vi "Sine Wave Generation.vi"() -> ()   [LabVIEW 2022 SP3]
uses:
  <instrlib>/niUSRP/niUSRP Write Tx Data (CDB).vi
panel:
  in  "Waveform size":i32
  out "coerced gain":dbl format="%#_6f"
  out "coerced carrier frequency":dbl=100000.0 format="%#_6p"
  out "coerced IQ rate":dbl=100000.0 format="%#_6p"
  in  "active antenna 2":string
  in  "gain (dB)":dbl
  in  "?":bool
  in  "frequency (Hz)":dbl
  in  "IQ rate (S/s)":dbl
  in  "USRP IP Address":refnum<k15>
  out "error out":errorcluster
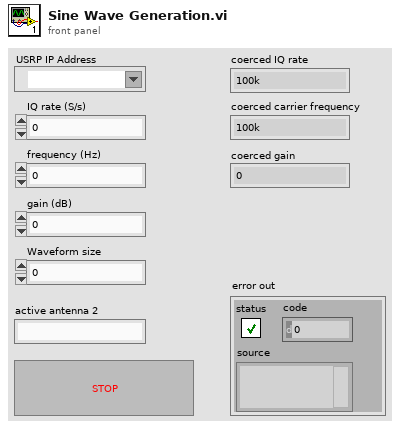
[diagram p1: front panel]
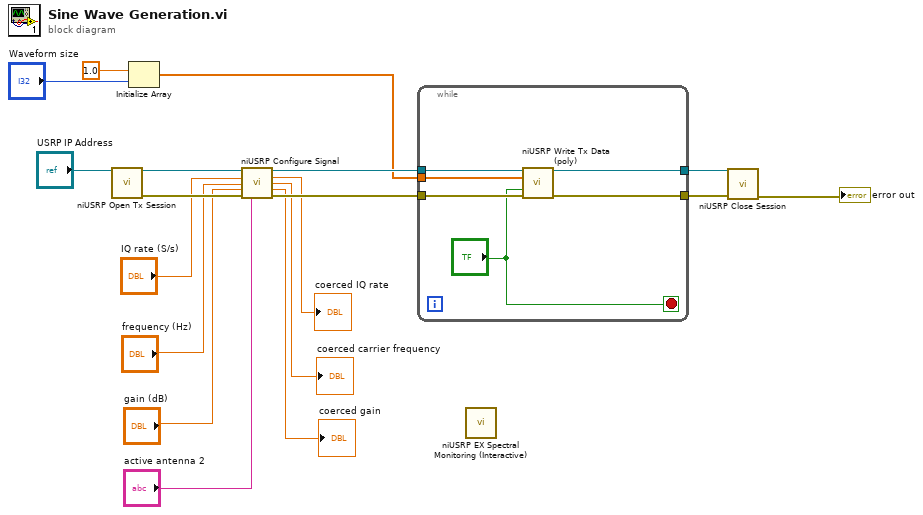
[diagram p0: block diagram]
diagram:
  n1 = call <instrlib>:"niUSRP Open Tx Session.vi"("device names"="USRP IP Address") -> ("session handle out"=w14:refnum<k15>, "error out"=w17:errorcluster)  [unwired: 13 in]
  n2 = Initialize Array(1.0, "Waveform size") -> (w2:dbl[])
  n3 = call <instrlib>:"niUSRP Configure Signal.vi"("session handle"=w14, "IQ rate"="IQ rate (S/s)", "carrier frequency"="frequency (Hz)", "gain"="gain (dB)", "error in (no error)"=w17, "active antenna"="active antenna 2") -> ("session handle out"=w13:refnum<k15>, "coerced IQ rate"=→"coerced IQ rate":dbl, "coerced carrier frequency"=→"coerced carrier frequency":dbl, "coerced gain"=→"coerced gain":dbl, "error out"=w16:errorcluster)  [unwired: 5 in]
  n4 = while {
    tunnel: w16 -> [w24]
    tunnel: [w23] -> w15
    tunnel: w13 -> [w22]
    tunnel: [w21] -> w12
    tunnel: w2 -> [w20]
    stop <- "?" stop-if-true
    n5 = call-poly <instrlib>:"niUSRP Write Tx Data (poly).vi"("session handle"=w22, "data"=w20, "end of data?"="?", "error in (no error)"=w24) -> ("session handle out"=w21:refnum<k15>, "error out"=w23:errorcluster)  [unwired: 10 in]
  }
  n6 = call "niUSRP EX Spectral Monitoring (Interactive).vi"() -> ()  [unwired: 1 in]
  n7 = call <instrlib>:"niUSRP Close Session.vi"("session handle"=w12, "error in (no error)"=w15) -> ("error out"=→"error out":errorcluster)  [unwired: 13 in]
